vi "Редактирование.vi"() -> ()   [LabVIEW 2017]
doc: "This VI is used in Exercise 2-2 of the LabVIEW Basics I Course. You follow the directions in the labels on the front panel to learn and practice editing techniques in LabVIEW."
uses:
  <vilib>/Analysis/NI_AALBase.lvlib
panel:
  out "Изменить размер  отдельного элемента\nотображения - лампы и изменить цвет \nсостояния OFF на зеленый, \nа состояния ON на красный":bool
  out "График Диаграмм. Изменить тип, рамер и цвет шрифта  \nи маштаб шкалы оси Y.":dbl[](graph)
  out "c":bool
  in  "A":bool
  in  "Цифрой элемент управления (собственная метка)\nИзменить положение.":dbl format="%.2f"
  out "?":dbl format="%.2f"
  in  "?":string="Строковый элемент управления."
  out "b":bool
  out "a":bool
  in  "B":bool
  in  "C":bool
  # "Создать собственную метку цифрового \nэлемента отображения."
  # "Свободная метка.\nСоздать копию."
  # "Изменить положение группы элементов - \n3-х переключателей (A, B,C)."
  # "Свободная метка. Изменить тип шрифта и скрыть \nконтур вокруг метки."
  # "Выровнить элементы индикаторов- \n3 лампы (a, b, c)  по  горизонтали и равномерно\n распределить пространство между ними."
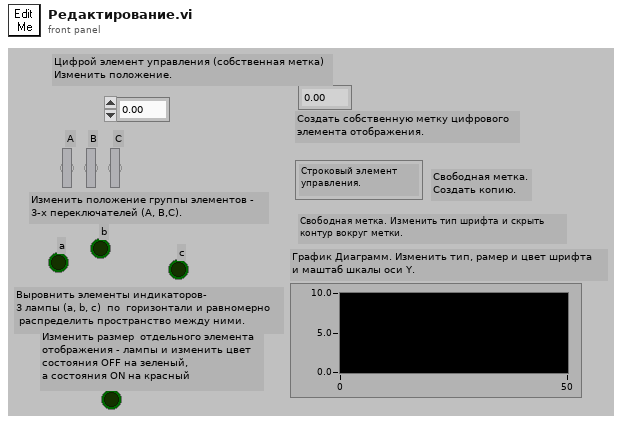
[diagram p1: front panel]
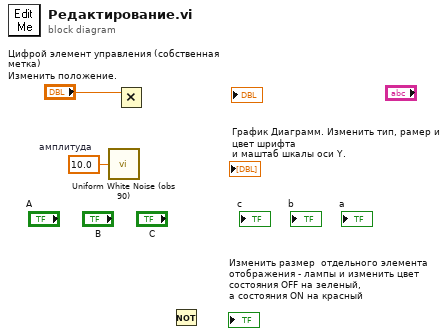
[diagram p0: block diagram]
diagram:
  w1 = 10.0  # амплитуда
  n1 = call <vilib>:"Uniform White Noise (obs 90).vi"("amplitude"=w1) -> ()  [unwired: 2 in, 2 out]
  n2 = Multiply(x="Цифрой элемент управления (собственная метка)\nИзменить положение.") -> ()  [unwired: 1 in, 1 out]
  n3 = Not() -> ()  [unwired: 1 in, 1 out]
